vi "SuperSimpleMotorTest.vi"() -> ()   [LabVIEW 2009]
uses:
  <vilib>/eio/EIONode/EIONode.xnode
  <vilib>/rvi/eio/nirviEIOImplementation/nirviEIOImplementation.xnode
  <vilib>/rvi/eio/common/nirviEmuTemplateMethod_noerrors.vi
  <vilib>/rvi/eio/common/nirviEmuClasses.ctl
panel:
  in  "stop":bool
  in  "M2 Enable":bool
  in  "M1 Enable":bool
  in  "M0 Enable":bool
  in  "M2 output":fxp<+/-,20,5>
  in  "M1 output":fxp<+/-,20,5>
  in  "M0 output":fxp<+/-,20,5>
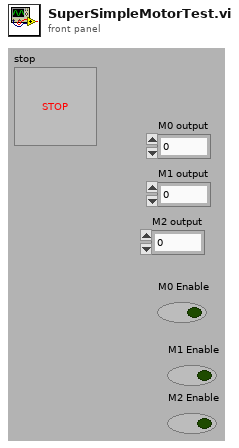
[diagram p1: front panel]
types:
  T1 = typedef "nirviEmuClasses.ctl" = enum16{"IO Read", "IO Write", "Method", "Property Read", "Property Write"}
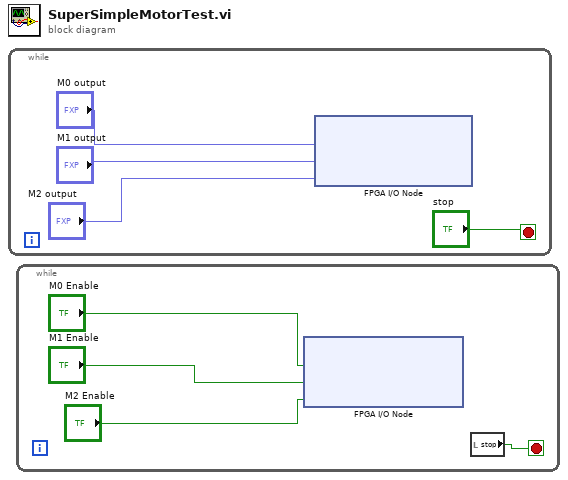
[diagram p0: block diagram]
diagram:
  n1 = while {
    stop <- "stop" stop-if-true
    n2 = xnode "FPGA I/O Node"("Drive Motor Speed"="M0 output", "Steering Motor Speed"="M1 output", "Lidar Motor Speed"="M2 output") -> ()  [unwired: 3 in, 3 out]
  }
  n3 = while {
    stop <- w38 stop-if-true
    n4 = xnode "FPGA I/O Node"("Drive Motor Inhibit"="M0 Enable", "Steering Motor Inhibit"="M1 Enable", "Lidar Motor Inhibit"="M2 Enable") -> ()  [unwired: 3 in, 3 out]
    n5 = local read "stop"() -> (w38:bool)
  }
